vi "Create All Data Queues.vi"(8 "Error In":errorcluster) -> (0 "Error Out":errorcluster, 3 "WINFAS 2 Data Queue.lvlib:All Data Queues Cluster":T1)   [LabVIEW 2014, in "WINFAS 2 Data Queue.lvlib"]
uses:
  WINFAS 2 Data Queue.lvlib
  All Data Queues Cluster.ctl
  Acquisition Data 1 Sample Cluster.ctl
  Control Data Cluster.ctl
  Async Acquisition Data Cluster.ctl
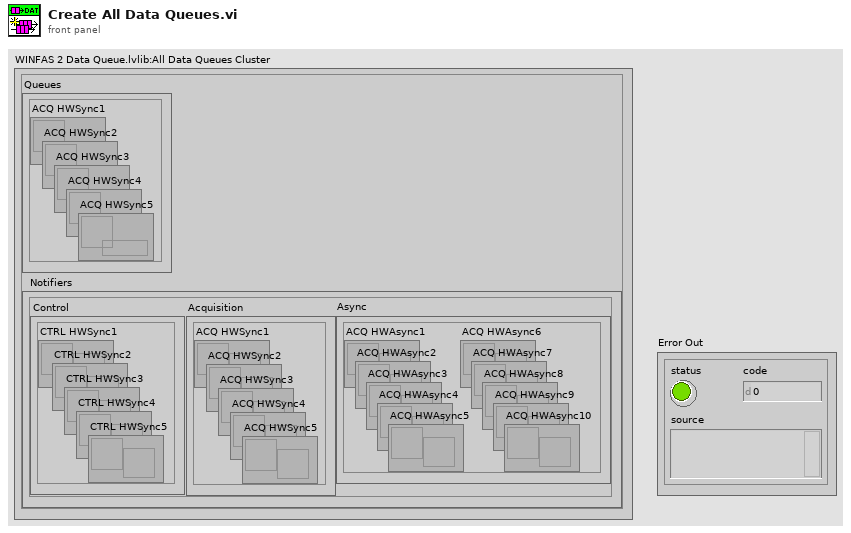
[diagram p1: front panel]
types:
  T1 = typedef "WINFAS 2 Data Queue.lvlib/All Data Queues Cluster.ctl" = cluster{"Queues":cluster{"ACQ HWSync1":refnum<queue>, "ACQ HWSync2":refnum<queue>, "ACQ HWSync3":refnum<queue>, "ACQ HWSync4":refnum<queue>, "ACQ HWSync5":refnum<queue>}, "Notifiers":cluster{"Control":cluster{"CTRL HWSync1":refnum<notifier>, "CTRL HWSync2":refnum<notifier>, "CTRL HWSync3":refnum<notifier>, "CTRL HWSync4":refnum<notifier>, "CTRL HWSync5":refnum<notifier>}, "Acquisition":cluster{"ACQ HWSync1":refnum<notifier>, "ACQ HWSync2":refnum<notifier>, "ACQ HWSync3":refnum<notifier>, "ACQ HWSync4":refnum<notifier>, "ACQ HWSync5":refnum<notifier>}, "Async":cluster{"ACQ HWAsync1":refnum<notifier>, "ACQ HWAsync2":refnum<notifier>, "ACQ HWAsync3":refnum<notifier>, "ACQ HWAsync4":refnum<notifier>, "ACQ HWAsync5":refnum<notifier>, "ACQ HWAsync6":refnum<notifier>, "ACQ HWAsync7":refnum<notifier>, "ACQ HWAsync8":refnum<notifier>, "ACQ HWAsync9":refnum<notifier>, "ACQ HWAsync10":refnum<notifier>}}}
  T2 = cluster{"Control":cluster{"CTRL HWSync1":refnum<notifier>, "CTRL HWSync2":refnum<notifier>, "CTRL HWSync3":refnum<notifier>, "CTRL HWSync4":refnum<notifier>, "CTRL HWSync5":refnum<notifier>}, "Acquisition":cluster{"ACQ HWSync1":refnum<notifier>, "ACQ HWSync2":refnum<notifier>, "ACQ HWSync3":refnum<notifier>, "ACQ HWSync4":refnum<notifier>, "ACQ HWSync5":refnum<notifier>}, "Async":cluster{"ACQ HWAsync1":refnum<notifier>, "ACQ HWAsync2":refnum<notifier>, "ACQ HWAsync3":refnum<notifier>, "ACQ HWAsync4":refnum<notifier>, "ACQ HWAsync5":refnum<notifier>, "ACQ HWAsync6":refnum<notifier>, "ACQ HWAsync7":refnum<notifier>, "ACQ HWAsync8":refnum<notifier>, "ACQ HWAsync9":refnum<notifier>, "ACQ HWAsync10":refnum<notifier>}}
  T3 = cluster{"ACQ HWSync1":refnum<queue>, "ACQ HWSync2":refnum<queue>, "ACQ HWSync3":refnum<queue>, "ACQ HWSync4":refnum<queue>, "ACQ HWSync5":refnum<queue>}
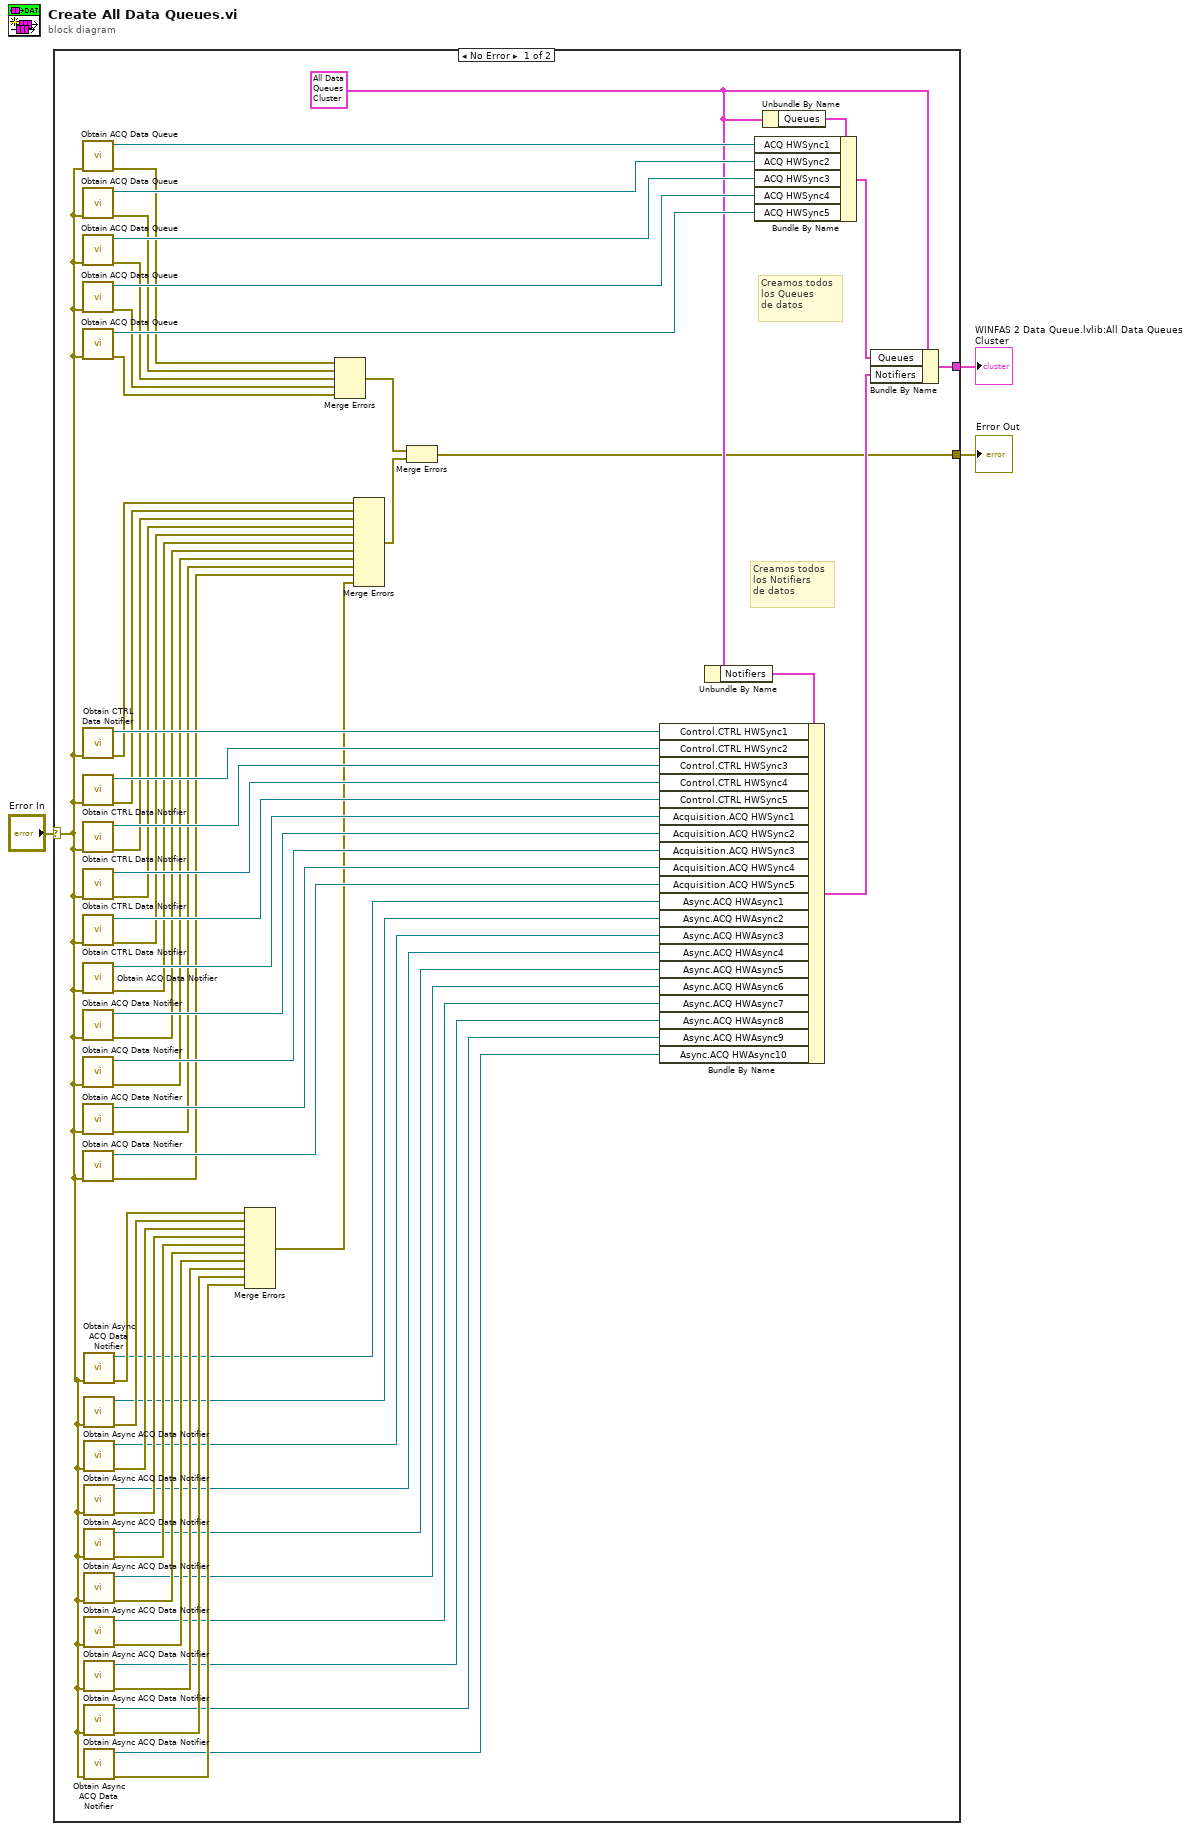
[diagram p0: block diagram]
diagram:
  n1 = case shown="No Error" "Error In" {
    selector: "Error In" -> [w4 w65]
    tunnel: [w32 w65] -> w2
    tunnel: [w64 _] -> w1
    frame No Error {
      w57 = T1 {"Queues"={"ACQ HWSync1"=refnum, "ACQ HWSync2"=refnum, "ACQ HWSync3"=refnum, "ACQ HWSync4"=refnum, "ACQ HWSync5"=refnum}, "Notifiers"={"Control"={"CTRL HWSync1"=refnum, "CTRL HWSync2"=refnum, "CTRL HWSync3"=refnum, "CTRL HWSync4"=refnum, "CTRL HWSync5"=refnum}, "Acquisition"={"ACQ HWSync1"=refnum, "ACQ HWSync2"=refnum, "ACQ HWSync3"=refnum, "ACQ HWSync4"=refnum, "ACQ HWSync5"=refnum}, "Async"={"ACQ HWAsync1"=refnum, "ACQ HWAsync2"=refnum, "ACQ HWAsync3"=refnum, "ACQ HWAsync4"=refnum, "ACQ HWAsync5"=refnum, "ACQ HWAsync6"=refnum, "ACQ HWAsync7"=refnum, "ACQ HWAsync8"=refnum, "ACQ HWAsync9"=refnum, "ACQ HWAsync10"=refnum}}} ("WINFAS 2 Data Queue.lvlib:All Data Queues Cluster")
      # "Creamos todos\nlos Notifiers\nde datos"
      # "Creamos todos\nlos Queues\nde datos"
      n2 = call "Obtain ACQ Data Queue.vi"("error in (no error)"=w4) -> ("error out"=w30:errorcluster, "ACQ Data Queue out"=w62:refnum<queue>)  [unwired: 9 in]
      n3 = call "Obtain ACQ Data Queue.vi"("error in (no error)"=w4) -> ("error out"=w29:errorcluster, "ACQ Data Queue out"=w61:refnum<queue>)  [unwired: 9 in]
      n4 = call "Obtain ACQ Data Queue.vi"("error in (no error)"=w4) -> ("error out"=w28:errorcluster, "ACQ Data Queue out"=w60:refnum<queue>)  [unwired: 9 in]
      n5 = call "Obtain ACQ Data Queue.vi"("error in (no error)"=w4) -> ("error out"=w27:errorcluster, "ACQ Data Queue out"=w59:refnum<queue>)  [unwired: 9 in]
      n6 = call "Obtain ACQ Data Queue.vi"("error in (no error)"=w4) -> ("error out"=w26:errorcluster, "ACQ Data Queue out"=w58:refnum<queue>)  [unwired: 9 in]
      n7 = call "Obtain CTRL Data Notifier.vi"("error in (no error)"=w4) -> ("error out"=w43:errorcluster, "CTRL Data Notifier out"=w55:refnum<notifier>)  [unwired: 9 in]
      n8 = call "Obtain CTRL Data Notifier.vi"("error in (no error)"=w4) -> ("error out"=w42:errorcluster, "CTRL Data Notifier out"=w54:refnum<notifier>)  [unwired: 9 in]
      n9 = call "Obtain CTRL Data Notifier.vi"("error in (no error)"=w4) -> ("error out"=w41:errorcluster, "CTRL Data Notifier out"=w53:refnum<notifier>)  [unwired: 9 in]
      n10 = call "Obtain CTRL Data Notifier.vi"("error in (no error)"=w4) -> ("error out"=w40:errorcluster, "CTRL Data Notifier out"=w52:refnum<notifier>)  [unwired: 9 in]
      n11 = call "Obtain CTRL Data Notifier.vi"("error in (no error)"=w4) -> ("error out"=w39:errorcluster, "CTRL Data Notifier out"=w51:refnum<notifier>)  [unwired: 9 in]
      n12 = call "Obtain ACQ Data Notifier.vi"("error in (no error)"=w4) -> ("error out"=w38:errorcluster, "ACQ Data Notifier out"=w50:refnum<notifier>)  [unwired: 9 in]
      n13 = call "Obtain ACQ Data Notifier.vi"("error in (no error)"=w4) -> ("error out"=w37:errorcluster, "ACQ Data Notifier out"=w49:refnum<notifier>)  [unwired: 9 in]
      n14 = call "Obtain ACQ Data Notifier.vi"("error in (no error)"=w4) -> ("error out"=w36:errorcluster, "ACQ Data Notifier out"=w48:refnum<notifier>)  [unwired: 9 in]
      n15 = call "Obtain ACQ Data Notifier.vi"("error in (no error)"=w4) -> ("error out"=w35:errorcluster, "ACQ Data Notifier out"=w47:refnum<notifier>)  [unwired: 9 in]
      n16 = call "Obtain ACQ Data Notifier.vi"("error in (no error)"=w4) -> ("error out"=w34:errorcluster, "ACQ Data Notifier out"=w46:refnum<notifier>)  [unwired: 9 in]
      n17 = call "Obtain Async ACQ Data Notifier.vi"("error in (no error)"=w4) -> ("error out"=w25:errorcluster, "Async ACQ Notifier out"=w15:refnum<notifier>)  [unwired: 9 in]
      n18 = call "Obtain Async ACQ Data Notifier.vi"("error in (no error)"=w4) -> ("error out"=w24:errorcluster, "Async ACQ Notifier out"=w13:refnum<notifier>)  [unwired: 9 in]
      n19 = call "Obtain Async ACQ Data Notifier.vi"("error in (no error)"=w4) -> ("error out"=w23:errorcluster, "Async ACQ Notifier out"=w12:refnum<notifier>)  [unwired: 9 in]
      n20 = call "Obtain Async ACQ Data Notifier.vi"("error in (no error)"=w4) -> ("error out"=w22:errorcluster, "Async ACQ Notifier out"=w11:refnum<notifier>)  [unwired: 9 in]
      n21 = call "Obtain Async ACQ Data Notifier.vi"("error in (no error)"=w4) -> ("error out"=w21:errorcluster, "Async ACQ Notifier out"=w10:refnum<notifier>)  [unwired: 9 in]
      n22 = call "Obtain Async ACQ Data Notifier.vi"("error in (no error)"=w4) -> ("error out"=w20:errorcluster, "Async ACQ Notifier out"=w9:refnum<notifier>)  [unwired: 9 in]
      n23 = call "Obtain Async ACQ Data Notifier.vi"("error in (no error)"=w4) -> ("error out"=w19:errorcluster, "Async ACQ Notifier out"=w8:refnum<notifier>)  [unwired: 9 in]
      n24 = call "Obtain Async ACQ Data Notifier.vi"("error in (no error)"=w4) -> ("error out"=w18:errorcluster, "Async ACQ Notifier out"=w7:refnum<notifier>)  [unwired: 9 in]
      n25 = call "Obtain Async ACQ Data Notifier.vi"("error in (no error)"=w4) -> ("error out"=w17:errorcluster, "Async ACQ Notifier out"=w6:refnum<notifier>)  [unwired: 9 in]
      n26 = call "Obtain Async ACQ Data Notifier.vi"("error in (no error)"=w4) -> ("error out"=w16:errorcluster, "Async ACQ Notifier out"=w5:refnum<notifier>)  [unwired: 9 in]
      n27 = Merge Errors(w25, w24, w23, w22, w21, w20, w19, w18, w17, w16) -> (w14:errorcluster)
      n28 = Merge Errors(w30, w29, w28, w27, w26) -> (w31:errorcluster)
      n29 = Merge Errors(w43, w42, w41, w40, w39, w38, w37, w36, w35, w34, w14) -> (w33:errorcluster)
      n30 = Merge Errors(w31, w33) -> (w32:errorcluster)
      n31 = Unbundle By Name(w57) -> ("Notifiers"=w56:T2)
      n32 = Bundle By Name(cluster=w56, "Control.CTRL HWSync1"=w55, "Control.CTRL HWSync2"=w54, "Control.CTRL HWSync3"=w53, "Control.CTRL HWSync4"=w52, "Control.CTRL HWSync5"=w51, "Acquisition.ACQ HWSync1"=w50, "Acquisition.ACQ HWSync2"=w49, "Acquisition.ACQ HWSync3"=w48, "Acquisition.ACQ HWSync4"=w47, "Acquisition.ACQ HWSync5"=w46, "Async.ACQ HWAsync1"=w15, "Async.ACQ HWAsync2"=w13, "Async.ACQ HWAsync3"=w12, "Async.ACQ HWAsync4"=w11, "Async.ACQ HWAsync5"=w10, "Async.ACQ HWAsync6"=w9, "Async.ACQ HWAsync7"=w8, "Async.ACQ HWAsync8"=w7, "Async.ACQ HWAsync9"=w6, "Async.ACQ HWAsync10"=w5) -> (w44:T2)
      n33 = Unbundle By Name(w57) -> ("Queues"=w63:T3)
      n34 = Bundle By Name(cluster=w63, "ACQ HWSync1"=w62, "ACQ HWSync2"=w61, "ACQ HWSync3"=w60, "ACQ HWSync4"=w59, "ACQ HWSync5"=w58) -> (w45:T3)
      n35 = Bundle By Name(cluster=w57, "Queues"=w45, "Notifiers"=w44) -> (w64:T1)
    }
    frame Error {
    }
  }
  "Error Out" <- w2
  "WINFAS 2 Data Queue.lvlib:All Data Queues Cluster" <- w1
